vi "bats.parser.test.AddOrderLong.add.two.tickers.vi"(10 "Expected OrderBook.Command[]":T2[](array[typedef])=[{"type"=enum."AddOrder", "side"=66, "orderId "=3544385890602799695, "quantity"=20000, "symbol"=4702127773838221344, "price"=9050, "executed.qty"=0, "canceled.qty"=0, "remaining.qty"=0, "seconds"=0, "nanoseconds"=447001, "Add"=FALSE, "Edit"=FALSE, "Remove"=FALSE, "seq no"=1, "recv.time"=0, "parse.time"=0}, {"type"=enum."AddOrder", "side"=66, "orderId "=3616443484640727631, "quantity"=20001, "symbol"=4702127773838221344, "price"=9050, "executed.qty"=0, "canceled.qty"=0, "remaining.qty"=0, "seconds"=0, "nanoseconds"=447002, "Add"=FALSE, "Edit"=FALSE, "Remove"=FALSE, "seq no"=2, "recv.time"=0, "parse.time"=0}, {"type"=enum."AddOrder", "side"=66, "orderId "=3688501078678655567, "quantity"=20002, "symbol"=6076284164848492576, "price"=9050, "executed.qty"=0, "canceled.qty"=0, "remaining.qty"=0, "seconds"=0, "nanoseconds"=447003, "Add"=FALSE, "Edit"=FALSE, "Remove"=FALSE, "seq no"=3, "recv.time"=0, "parse.time"=0}, {"type"=enum."AddOrder", "side"=66, "orderId "=3760558672716583503, "quantity"=20000, "symbol"=4702127773838213120, "price"=9050, "executed.qty"=0, "canceled.qty"=0, "remaining.qty"=0, "seconds"=0, "nanoseconds"=0, "Add"=FALSE, "Edit"=FALSE, "Remove"=FALSE, "seq no"=0, "recv.time"=0, "parse.time"=0}, {"type"=enum."AddOrder", "side"=66, "orderId "=3832616266754511439, "quantity"=20000, "symbol"=4702127773838213120, "price"=9050, "executed.qty"=0, "canceled.qty"=0, "remaining.qty"=0, "seconds"=0, "nanoseconds"=0, "Add"=FALSE, "Edit"=FALSE, "Remove"=FALSE, "seq no"=0, "recv.time"=0, "parse.time"=0}, {"type"=enum."AddOrder", "side"=66, "orderId "=3904673860792439375, "quantity"=20000, "symbol"=4702127773838213120, "price"=9050, "executed.qty"=0, "canceled.qty"=0, "remaining.qty"=0, "seconds"=0, "nanoseconds"=0, "Add"=FALSE, "Edit"=FALSE, "Remove"=FALSE, "seq no"=0, "recv.time"=0, "parse.time"=0}, {"type"=enum."AddOrder", "side"=66, "orderId "=3976731454830367311, "quantity"=20000, "symbol"=4702127773838213120, "price"=9050, "executed.qty"=0, "canceled.qty"=0, "remaining.qty"=0, "seconds"=0, "nanoseconds"=0, "Add"=FALSE, "Edit"=FALSE, "Remove"=FALSE, "seq no"=0, "recv.time"=0, "parse.time"=0}, {"type"=enum."AddOrder", "side"=66, "orderId "=4048789048868295247, "quantity"=20000, "symbol"=4702127773838213120, "price"=9050, "executed.qty"=0, "canceled.qty"=0, "remaining.qty"=0, "seconds"=0, "nanoseconds"=0, "Add"=FALSE, "Edit"=FALSE, "Remove"=FALSE, "seq no"=0, "recv.time"=0, "parse.time"=0}, {"type"=enum."AddOrder", "side"=66, "orderId "=4120846642906223183, "quantity"=20000, "symbol"=4702127773838213120, "price"=9050, "executed.qty"=0, "canceled.qty"=0, "remaining.qty"=0, "seconds"=0, "nanoseconds"=0, "Add"=FALSE, "Edit"=FALSE, "Remove"=FALSE, "seq no"=0, "recv.time"=0, "parse.time"=0}, {"type"=enum."AddOrder", "side"=66, "orderId "=4697307395209646671, "quantity"=20000, "symbol"=4702127773838213120, "price"=9050, "executed.qty"=0, "canceled.qty"=0, "remaining.qty"=0, "seconds"=0, "nanoseconds"=0, "Add"=FALSE, "Edit"=FALSE, "Remove"=FALSE, "seq no"=0, "recv.time"=0, "parse.time"=0}, {"type"=enum."AddOrder", "side"=66, "orderId "=4769364989247574607, "quantity"=20000, "symbol"=4702127773838213120, "price"=9050, "executed.qty"=0, "canceled.qty"=0, "remaining.qty"=0, "seconds"=0, "nanoseconds"=0, "Add"=FALSE, "Edit"=FALSE, "Remove"=FALSE, "seq no"=0, "recv.time"=0, "parse.time"=0}] {"symbol" format="%.0x"; "orderId" format="%.0x"; "side" format="%.0x"}) -> ()   [LabVIEW 2020]
uses:
  Market.Data.Common/fpga/orderbook.command.ctl
  Market.Data.Common/fpga/orderbook.command.type.ctl
  pitch/AddOrder/AddOrderLong.Parameters.ctl
  Market.Data.Common/fpga/fpganow.common.fpga.lvlib
  pitch/AddOrder/AddOrderLong.lvclass
panel:
  out "Passed":bool
  in  "AddOrderLong.Parameters 3":T1={"Time Offset"=447003, "Order Id"="ORID0003", "Quantity"=20002, "Symbol"="TSLA", "Side Indicator"="B", "Price"=0.905}
  in  "AddOrderLong.Parameters 2":T1={"Time Offset"=447002, "Order Id"="ORID0002", "Quantity"=20001, "Symbol"="AAPL", "Side Indicator"="B", "Price"=0.905}
  in  "AddOrderLong.Parameters":T1={"Time Offset"=447001, "Order Id"="ORID0001", "Quantity"=20000, "Symbol"="AAPL", "Side Indicator"="B", "Price"=0.905}
  out "Debug":u64[](array[numeric]) format="%.0x"
  out "Results":T2[](array[typedef]) {"symbol" format="%.0x"; "orderId" format="%.0x"; "side" format="%.0x"}
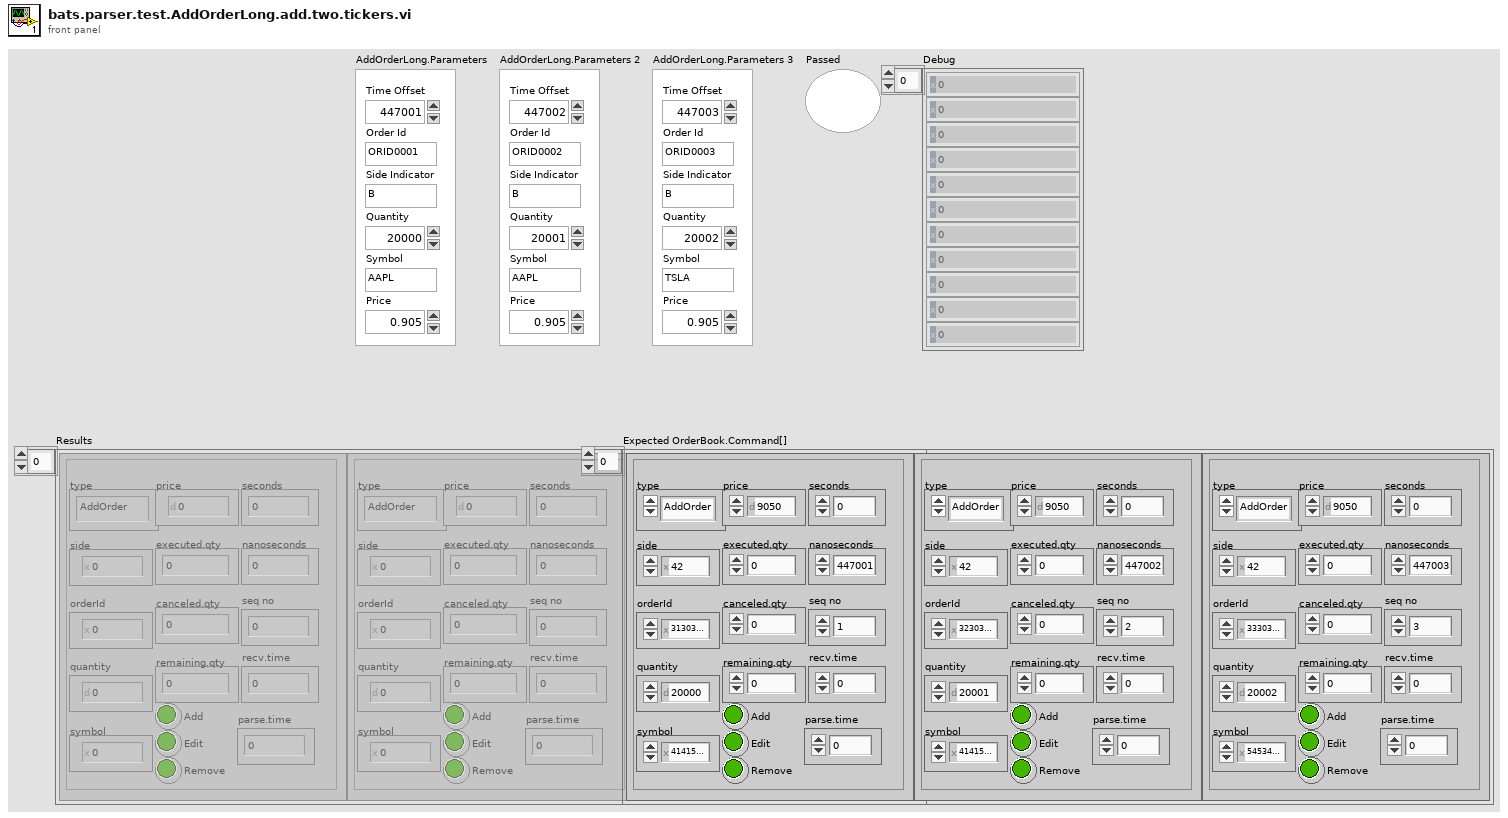
[diagram p1: front panel]
types:
  T1 = typedef "AddOrderLong.lvclass/AddOrderLong.Parameters.ctl" = cluster{"Time Offset":u32, "Order Id":string, "Quantity":u32, "Symbol":string, "Side Indicator":string, "Price":dbl}
  T2 = typedef "fpganow.common.fpga.lvlib/orderbook.command.ctl" = cluster{"type":T3, "side":u8, "orderId ":u64, "quantity":u32, "symbol":u64, "price":u64, "executed.qty":u32, "canceled.qty":u32, "remaining.qty":u32, "seconds":u64, "nanoseconds":u64, "Add":bool, "Edit":bool, "Remove":bool, "seq no":u32, "recv.time":u64, "parse.time":u64}
  T3 = typedef "fpganow.common.fpga.lvlib/orderbook.command.type.ctl" = enum8{"Time", "AddOrder", "OrderExecuted", "OrderExecutedAtPrice", "ReduceSize", "ModifyOrder", "DeleteOrder", "Get.Everything", "Get.All.Orders", "Get.Top"}
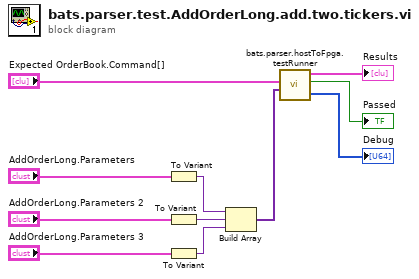
[diagram p0: block diagram]
diagram:
  n1 = To Variant(anything="AddOrderLong.Parameters") -> (Variant=w2:variant)
  n2 = To Variant(anything="AddOrderLong.Parameters 2") -> (Variant=w3:variant)
  n3 = To Variant(anything="AddOrderLong.Parameters 3") -> (Variant=w4:variant)
  n4 = Build Array(w2, w3, w4) -> (w1:variant[])
  n5 = call "bats.parser.hostToFpga.testRunner.vi"("Test.Messages"=w1, "Expected OrderBook.Command[]"="Expected OrderBook.Command[]") -> ("Passed"=→"Passed":bool, "OrderBook.Command[]"=→"Results":T2[], "Debug"=→"Debug":u64[])  [unwired: 4 in, 3 out]
